vi "LinxDigitalGetNumChans.vi"(8 "Error In":errorcluster, 11 "LINX Resource":T1) -> (0 "Error Out":errorcluster, 2 "DigitalNumChans":u8, 3 "LINX Resource":T1)   [LabVIEW 2014, in "LMH-LINX.lvlib" / "Local IO.lvlib"]
uses:
  <vilib>/MakerHub/LINX/Private/Local IO/Local IO.lvlib
  <vilib>/MakerHub/LINX/Private/Type Defs/LINX Ref.ctl
  <vilib>/MakerHub/LINX/Private/Type Defs/Platform.ctl
  <vilib>/MakerHub/LINX/Private/Type Defs/Interface.ctl
  <vilib>/MakerHub/LINX/Private/Device/Type Defs/LINX Device Config.ctl
  <vilib>/MakerHub/LINX/Private/Device/Type Defs/TCP Config.ctl
  <vilib>/MakerHub/LINX/Private/Device/Type Defs/Channels.ctl
  liblinxdevice.dll
  <vilib>/MakerHub/LINX/LMH-LINX.lvlib
  <vilib>/MakerHub/LINX/Private/Device/Device.lvlib
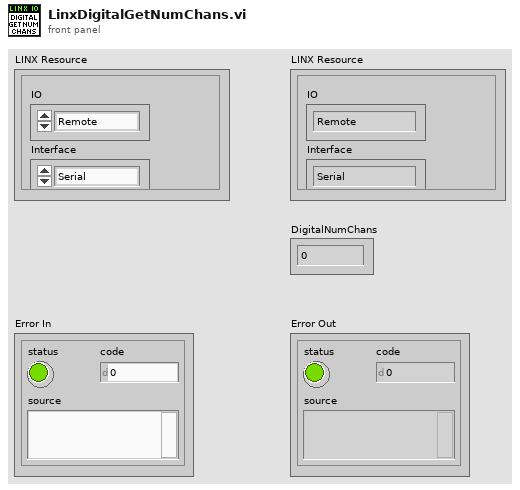
[diagram p1: front panel]
types:
  T1 = typedef "LMH-LINX.lvlib/LINX Ref.ctl" = cluster{"IO":T2, "Interface":T3, "LINX Device Config":T4}
  T2 = typedef "LMH-LINX.lvlib/Platform.ctl" = enum16{"Remote", "Local"}
  T3 = typedef "LMH-LINX.lvlib/Interface.ctl" = enum16{"Serial", "TCP"}
  T4 = typedef "LMH-LINX.lvlib/Device.lvlib/LINX Device Config.ctl" = cluster{"Interface":T3, "COM Port":refnum<visa-resource-name>, "TCP Configuration":T5, "Device Family":u8, "Device ID":u8, "Device Name":string, "TCP Ref":refnum<k5>, "Channels":T6}
  T5 = typedef "LMH-LINX.lvlib/Device.lvlib/TCP Config.ctl" = cluster{"IP Address":string, "Port":u16}
  T6 = typedef "LMH-LINX.lvlib/Channels.ctl" = cluster{"DI":u8[], "DO":u8[], "AI":u8[], "AO":u8[], "PWM":u8[], "QE":u8[], "UART":u8[], "I2C 2":u8[], "SPI":u8[], "CAN":u8[], "Servo":u8[], "AI Ref (V)":dbl, "AI Resolution (Bits)":u8, "AO Ref (V)":dbl, "AO Resolution (Bits)":u8}
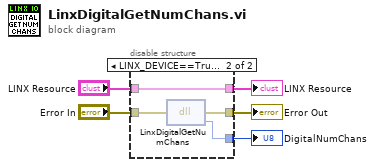
[diagram p0: block diagram]
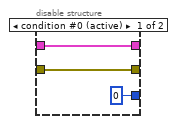
[diagram p2: hidden frame]
diagram:
  n1 = disable-structure shown="LINX_DEVICE==True" {
    disable-tunnel: "Error In" -> [w7 w12]
    disable-tunnel: [w7 w11] -> w4
    disable-tunnel: [u8 0 ("DigitalNumChans") w10] -> w3
    disable-tunnel: [w8 w9] -> w2
    disable-tunnel: "LINX Resource" -> [w8 w9]
    frame condition #0 (active) {
    }
    frame condition #1 {
      n2 = dll-call lib="liblinxdevice.*" fn="LinxDigitalGetNumChans"(error in=w12) -> (error out=w11:errorcluster, "DigitalNumChans"=w10:u8)  [unwired: 2 in, 1 out]
    }
  }
  "Error Out" <- w4
  "LINX Resource" <- w2
  "DigitalNumChans" <- w3
